vi "convert scan cluster to file scan.vi"(10 "precision (12)":i16=12, 11 "Scan parameters":T1 {"Scan Start" format="%#.9p"; "Scan End" format="%#.9p"; "Scan Step Size" format="%#.9p"}) -> (1 "values:numshots":string[](array[string]), 2 "values":string[](array[string]), 3 "spreadsheet string":string)   [LabVIEW 2013]
uses:
  scan parameters.ctl
  <vilib>/Analysis/1siggen.llb/Ramp Pattern by Delta.vi
  <vilib>/Analysis/NI_AALBase.lvlib
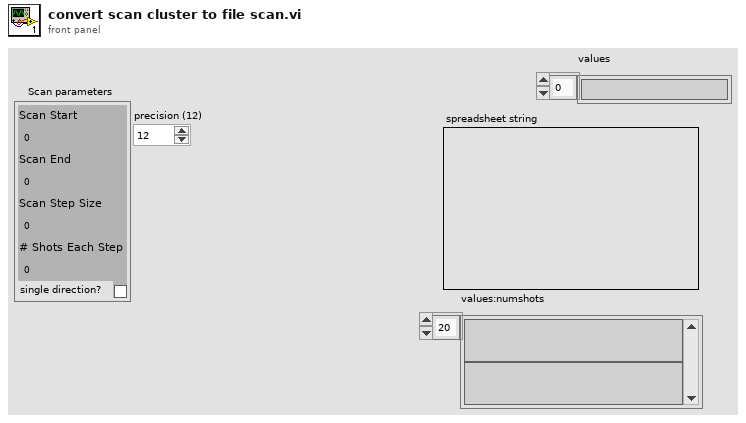
[diagram p1: front panel]
types:
  T1 = typedef "scan parameters.ctl" = cluster{"Scan Start":dbl, "Scan End":dbl, "Scan Step Size":dbl, "# Shots Each Step":u32, "single direction?":bool}
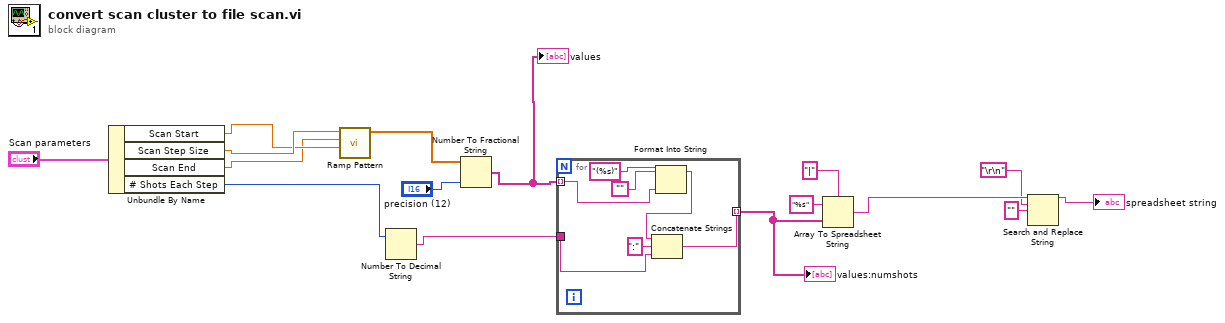
[diagram p0: block diagram]
diagram:
  n1 = Unbundle By Name("Scan parameters") -> ("Scan Start"=w14:dbl, "Scan Step Size"=w15:dbl, "Scan End"=w13:dbl, "# Shots Each Step"=w10:u32)
  n2 = call-poly <vilib>:"Ramp Pattern.vi"("start"=w14, "end"=w13, "delta"=w15) -> ("Ramp Pattern"=w11:dbl[])  [unwired: 6 in, 2 out]
  n3 = Number To Decimal String(number=w10) -> (decimal integer string=w9:string)  [unwired: 1 in]
  n4 = Number To Fractional String(number=w11, precision (6)="precision (12)") -> (F-format string=w5:string[])  [unwired: 2 in]
  "values" <- w5
  n5 = for {
    tunnel: w5 -> [w18] mode=indexing
    tunnel: w9 -> [w22]
    tunnel: [w21] -> w8 mode=indexing
    n6 = Format Into String(format string="(%s)", initial string="", w18) -> (resulting string=w17:string)  [unwired: 1 in, 1 out]
    n7 = Concatenate Strings(w17, ":" ("string"), w22) -> (w21:string)
  }
  "values:numshots" <- w8
  n8 = Array To Spreadsheet String(delimiter (Tab)="|", array=w8, 3:"%s" ("format string")) -> (spreadsheet string=w4:string)
  n9 = Search and Replace String(input string=w4, search string="\r\n", replace string="" ("replace string (\"\")")) -> (result string=→"spreadsheet string":string)  [unwired: 5 in, 3 out]
